vi "project 1.vi"() -> ()   [LabVIEW 2017]
uses:
  <vilib>/Instr/_visa.llb/VISA Configure Serial Port (Instr).vi
panel:
  in  "stop bits (10: 1 bit)":u16(ring)=10 items=["1.0"=10, "1.5"=15, "2.0"=20]
  in  "read":bool
  in  "delay before read":u32
  in  "write":bool
  out "?":u8
  out "Tank 2":u8(slide) scale=0.0..300.0
  out "Tank":u8(slide) scale=0.0..300.0
  out "Meter 2":u8(knob) scale=0.0..300.0
  out "Meter":u8(knob) scale=0.0..300.0
  out "output":bool[](array[boolean])
  out "?":u8
  out "string":string
  in  "Slide":u8(slide) scale=0.0..300.0
  in  "Array":bool[](array[boolean])
  in  "data bits (8)":u16=8 min=5 max=8 step=1
  in  "baud rate (9600)":u32=9600
  in  "VISA resource name":refnum<visa-resource-name>
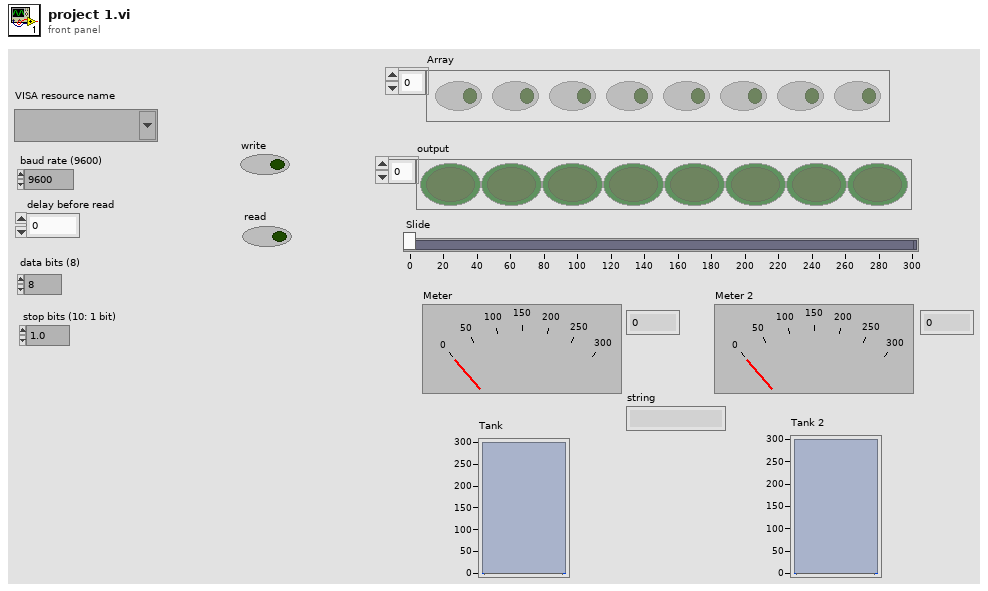
[diagram p1: front panel]
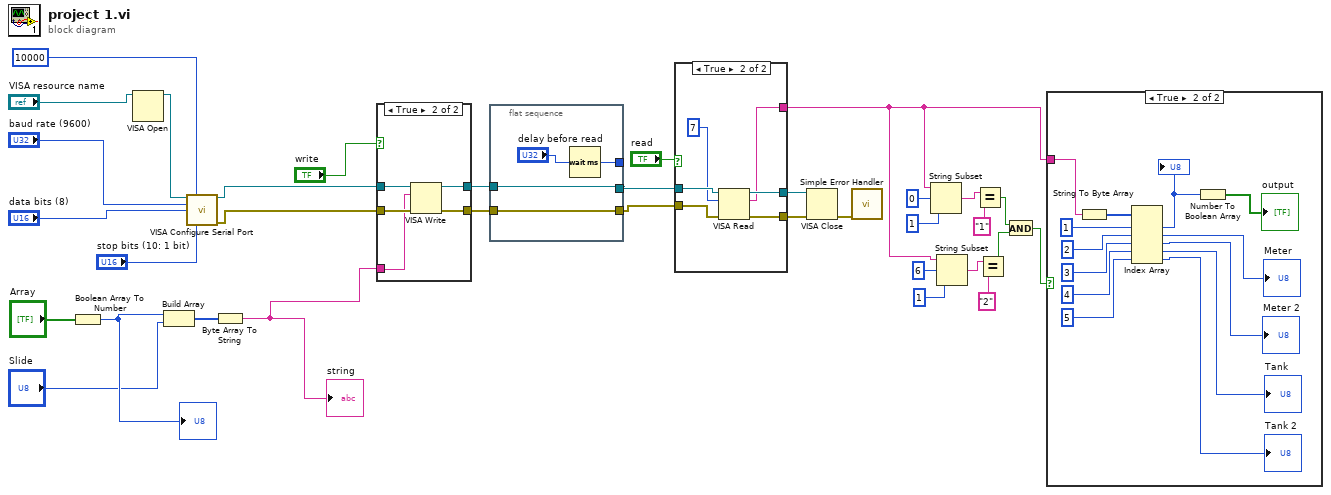
[diagram p0: block diagram]
diagram:
  n1 = Boolean Array To Number(Boolean array="Array") -> (number=w4:u32)
  "?" <- w4
  n2 = VISA Open(VISA resource name="VISA resource name") -> (VISA resource name=w1:refnum<visa-resource-name>)  [unwired: 4 in, 1 out]
  n3 = Build Array(w4, "Slide") -> (w5:u32[])
  n4 = call-poly "VISA Configure Serial Port"("VISA resource name"=w1, "timeout (10sec)"=u32 10000, "baud rate (9600)"="baud rate (9600)", "data bits (8)"="data bits (8)", "stop bits (10: 1 bit)"="stop bits (10: 1 bit)") -> ("VISA resource name out"=w17:refnum<visa-resource-name>, "error out"=w16:errorcluster)  [unwired: 9 in]
  n5 = Byte Array To String(unsigned byte array=w5) -> (string=w15:string)
  "string" <- w15
  n6 = case shown="True" "write" {
    tunnel: w17 -> [_ w39]
    tunnel: w16 -> [_ w38]
    tunnel: w15 -> [_ w37]
    tunnel: [_ w36] -> w13
    tunnel: [_ w35] -> w12
    frame False {
    }
    frame True {
      n7 = VISA Write(VISA resource name=w39, write buffer=w37, error in (no error)=w38) -> (VISA resource name out=w36:refnum<visa-resource-name>, error out=w35:errorcluster)  [unwired: 1 out]
    }
  }
  n8 = flat-sequence {
    tunnel: [w42] -> w10
    tunnel: w13 -> [w42]
    tunnel: [w41] -> w11
    tunnel: w12 -> [w41]
    tunnel: [w40] -> _
    frame #0 {
      n9 = Wait (ms)(milliseconds to wait="delay before read") -> (millisecond timer value=w40:u32)
    }
  }
  n10 = case shown="True" "read" {
    tunnel: [_ w47] -> w31
    tunnel: [_ w46] -> w30
    tunnel: w11 -> [_ w49]
    tunnel: w10 -> [_ w48]
    tunnel: [_ w44] -> w8
    frame False {
    }
    frame True {
      n11 = VISA Read(VISA resource name=w48, byte count=u32 7, error in (no error)=w49) -> (VISA resource name out=w47:refnum<visa-resource-name>, read buffer=w44:string, error out=w46:errorcluster)  [unwired: 1 out]
    }
  }
  n12 = VISA Close(VISA resource name=w31, error in (no error)=w30) -> (error out=w6:errorcluster)
  n13 = call <vilib>:"Simple Error Handler.vi"("error in (no error)"=w6) -> ()  [unwired: 4 in, 5 out]
  n14 = String Subset(string=w8, offset (0)=0, length (rest)=1 ("length (rest)")) -> (substring=w24:string)
  n15 = String Subset(string=w8, offset (0)=6, length (rest)=1 ("length (rest)")) -> (substring=w25:string)
  n16 = Equal?(x=w24, y="1") -> (x = y?=w21:bool)
  n17 = Equal?(x=w25, y="2") -> (x = y?=w20:bool)
  n18 = And(x=w21, y=w20) -> (x .and. y?=w19:bool)
  n19 = case shown="True" w19 {
    tunnel: w8 -> [_ w62]
    frame False {
    }
    frame True {
      n20 = String To Byte Array(string=w62) -> (unsigned byte array=w61:u8[])
      n21 = Index Array(array=w61, index #1=1 ("index"), index #2=2 ("index"), index #3=3 ("index"), index #4=4 ("index"), index #5=5 ("index")) -> (element #1=w54:u8, element #2=→"Meter":u8, element #3=→"Meter 2":u8, element #4=→"Tank":u8, element #5=→"Tank 2":u8)
      "?" <- w54
      n22 = Number To Boolean Array(number=w54) -> (Boolean array=→"output":bool[])
    }
  }
